vi "Calculate X Parameters (SubVI).vi"(10 "Camera":i32[][](array[numeric]), 11 "DMD":i32[][](array[numeric])) -> (0 "Intercept Rate":dbl format="%_6f", 1 "Intercept":dbl format="%_6f", 2 "Slope Rate":dbl format="%_6f", 3 "Slope":dbl format="%_6f")   [LabVIEW 2017]
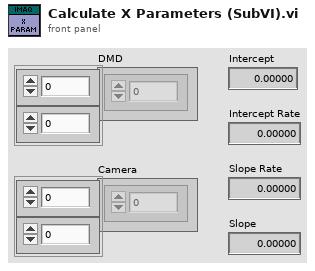
[diagram p1: front panel]
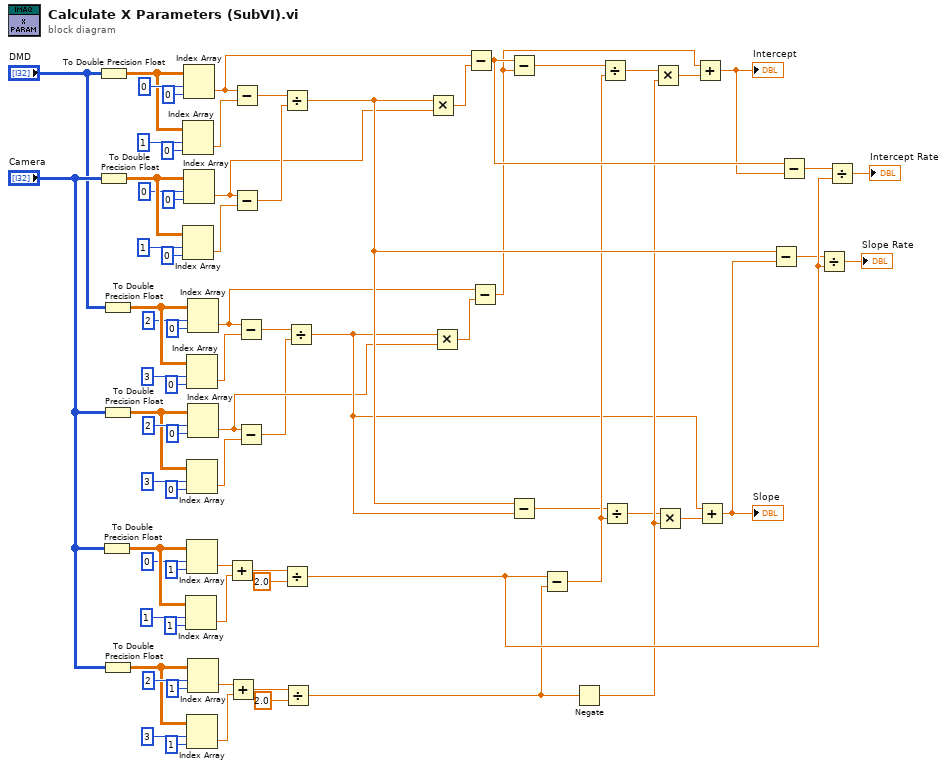
[diagram p0: block diagram]
diagram:
  n1 = To Double Precision Float(number="DMD") -> (double precision float=w13:dbl[][])
  n2 = To Double Precision Float(number="Camera") -> (double precision float=w10:dbl[][])
  n3 = To Double Precision Float(number="Camera") -> (double precision float=w39:dbl[][])
  n4 = To Double Precision Float(number="DMD") -> (double precision float=w22:dbl[][])
  n5 = To Double Precision Float(number="Camera") -> (double precision float=w25:dbl[][])
  n6 = To Double Precision Float(number="Camera") -> (double precision float=w49:dbl[][])
  n7 = Index Array(array=w13, index (row)=1, index (col)=0 ("disabled index (col)")) -> (element=w12:dbl)
  n8 = Index Array(array=w10, index (row)=1, index (col)=0 ("disabled index (col)")) -> (element=w11:dbl)
  n9 = Index Array(array=w13, index (row)=0, index (col)=0 ("disabled index (col)")) -> (element=w1:dbl)
  n10 = Index Array(array=w10, index (row)=0, index (col)=0 ("disabled index (col)")) -> (element=w3:dbl)
  n11 = Index Array(array=w39, index (row)=1, index (col)=1 ("disabled index (col)")) -> (element=w42:dbl)
  n12 = Index Array(array=w22, index (row)=3, index (col)=0 ("disabled index (col)")) -> (element=w23:dbl)
  n13 = Index Array(array=w25, index (row)=3, index (col)=0 ("disabled index (col)")) -> (element=w24:dbl)
  n14 = Index Array(array=w39, index (row)=0, index (col)=1 ("disabled index (col)")) -> (element=w41:dbl)
  n15 = Index Array(array=w49, index (row)=3, index (col)=1 ("disabled index (col)")) -> (element=w47:dbl)
  n16 = Index Array(array=w22, index (row)=2, index (col)=0 ("disabled index (col)")) -> (element=w34:dbl)
  n17 = Index Array(array=w25, index (row)=2, index (col)=0 ("disabled index (col)")) -> (element=w32:dbl)
  n18 = Index Array(array=w49, index (row)=2, index (col)=1 ("disabled index (col)")) -> (element=w48:dbl)
  n19 = Add(x=w41, y=w42) -> (x+y=w43:dbl)
  n20 = Add(x=w48, y=w47) -> (x+y=w46:dbl)
  n21 = Subtract(x=w1, y=w12) -> (x-y=w4:dbl)
  n22 = Subtract(x=w3, y=w11) -> (x-y=w5:dbl)
  n23 = Subtract(x=w34, y=w23) -> (x-y=w31:dbl)
  n24 = Subtract(x=w32, y=w24) -> (x-y=w30:dbl)
  n25 = Divide(x=w4, y=w5) -> (x/y=w64:dbl)
  n26 = Divide(x=w43, y=2.0) -> (x/y=w73:dbl)
  n27 = Divide(x=w46, y=2.0) -> (x/y=w70:dbl)
  n28 = Divide(x=w31, y=w30) -> (x/y=w58:dbl)
  n29 = Multiply(x=w64, y=w3) -> (x*y=w2:dbl)
  n30 = Multiply(x=w58, y=w32) -> (x*y=w33:dbl)
  n31 = Subtract(x=w1, y=w2) -> (x-y=w74:dbl)
  n32 = Subtract(x=w34, y=w33) -> (x-y=w63:dbl)
  n33 = Subtract(x=w74, y=w63) -> (x-y=w71:dbl)
  n34 = Subtract(x=w64, y=w58) -> (x-y=w55:dbl)
  n35 = Subtract(x=w73, y=w70) -> (x-y=w61:dbl)
  n36 = Negate(x=w70) -> (-x=w62:dbl)
  n37 = Divide(x=w71, y=w61) -> (x/y=w60:dbl)
  n38 = Divide(x=w55, y=w61) -> (x/y=w56:dbl)
  n39 = Multiply(x=w60, y=w62) -> (x*y=w59:dbl)
  n40 = Multiply(x=w56, y=w62) -> (x*y=w57:dbl)
  n41 = Add(x=w63, y=w59) -> (x+y=w72:dbl)
  "Intercept" <- w72
  n42 = Add(x=w58, y=w57) -> (x+y=w65:dbl)
  "Slope" <- w65
  n43 = Subtract(x=w64, y=w65) -> (x-y=w66:dbl)
  n44 = Subtract(x=w74, y=w72) -> (x-y=w69:dbl)
  n45 = Divide(x=w66, y=w73) -> (x/y=→"Slope Rate":dbl)
  n46 = Divide(x=w69, y=w73) -> (x/y=→"Intercept Rate":dbl)
